vi "Find Names.vi"(10 "Type Name Library File Path":T2) -> (1 "Name Library File Path":T1, 2 "Names":string[](array[string]))   [LabVIEW 2025, in "_Msg Rescript.lvlib" / "_Msg Rescript.lvclass"]
uses:
  _Msg Rescript.lvclass
  _Shared/Type Name Library File Path.ctl
  _Shared/Type.ctl
  _Shared/Name Library File Path.ctl
  _Msg Rescript.lvclass/_Msg Rescript.ctl
  _Shared/_Shared.lvlib
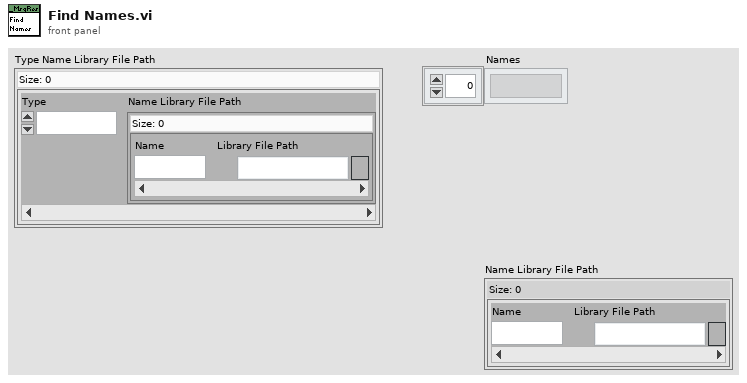
[diagram p1: front panel]
types:
  T1 = typedef "_Shared.lvlib/Name Library File Path.ctl" = map{string, path}
  T2 = typedef "_Shared.lvlib/Type Name Library File Path.ctl" = map{T3, T1}
  T3 = typedef "_Shared.lvlib/Type.ctl" = enum16{"Actor", "Msg"}
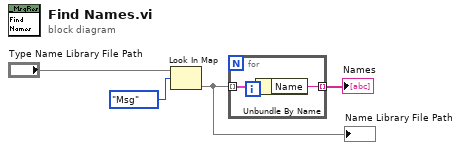
[diagram p0: block diagram]
diagram:
  n1 = Look In Map(map="Type Name Library File Path", key=Type."Msg" ("Type")) -> (value=w3:T1)  [unwired: 1 in, 1 out]
  "Name Library File Path" <- w3
  n2 = for {
    tunnel: w3 -> [w6] mode=indexing
    tunnel: [w5] -> w1 mode=indexing
    n3 = Unbundle By Name(w6) -> ("Name"=w5:string)
  }
  "Names" <- w1
